vi "FPGA - Finite Acq Engine.vi"(6 "Test Samples":u32, 9 "Last Iteraction Samples Acq":u32, 10 "Continue Test?":bool, 11 "Start Test?":bool) -> (1 "Samples Acq":u32, 2 "Continue Test":bool, 3 "Sample?":bool)   [LabVIEW 2012]
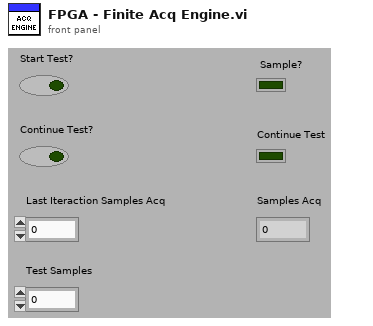
[diagram p1: front panel]
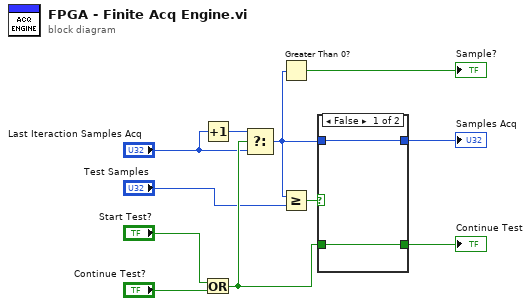
[diagram p0: block diagram]
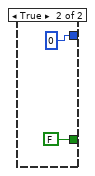
[diagram p2: hidden frame]
diagram:
  n1 = Increment(x="Last Iteraction Samples Acq") -> (x+1=w2:u32)
  n2 = Or(x="Start Test?", y="Continue Test?") -> (x .or. y?=w6:bool)
  n3 = Select(t=w2, s=w6, f="Last Iteraction Samples Acq") -> (s? t:f=w7:u32)
  n4 = Greater Than 0?(x=w7) -> (x > 0?=→"Sample?":bool)
  n5 = Greater Or Equal?(x=w7, y="Test Samples") -> (x >= y?=w9:bool)
  n6 = case shown="False" w9 {
    tunnel: w6 -> [w12 _]
    tunnel: w7 -> [w13 _]
    tunnel: [w13 u32 0 ("t")] -> w10
    tunnel: [w12 FALSE ("t")] -> w11
    frame False {
    }
    frame True {
    }
  }
  "Continue Test" <- w11
  "Samples Acq" <- w10
